vi "Get Section.vi"(10 "sections":string[](array[string]), 11 "info data":string) -> (1 "exist":bool, 3 "section part":string)   [LabVIEW 2013, in "infolib.lvlib"]
doc: "Finds section structure and return its content. If not found, exist is false. If no section structure set, returns whole info data and exist is true."
uses:
  infolib.lvlib
  <vilib>/regexp/Match Regular Expression.xnode
panel:
  out "element":string
  out "regexp":string
  # "testing string: (put \"1\" and \"2\" into section names)"
  # "blfdablad\n#startsection:: 1\njfkdla\n#startsection:: 2\ngroup2group2\n\t  \t#endsection:: 2\njdfkls\n#endsection:: 1\njfdklajfkdl"
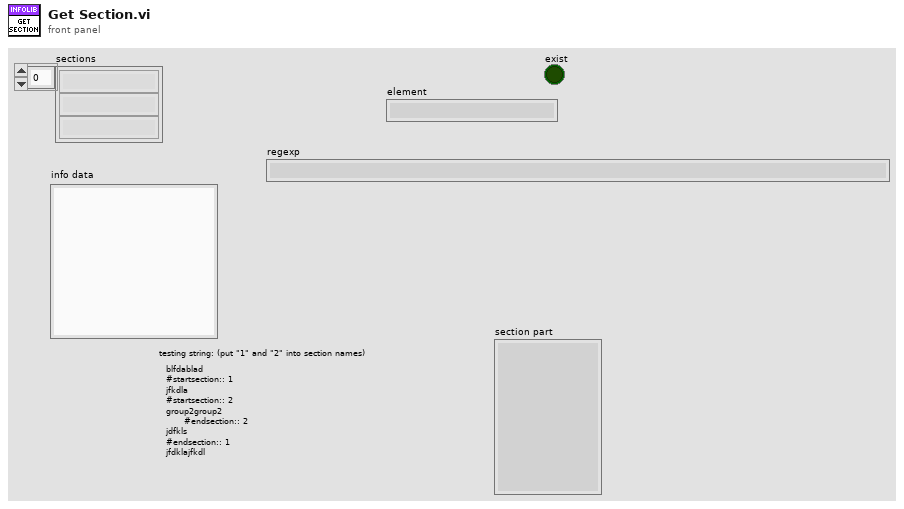
[diagram p1: front panel]
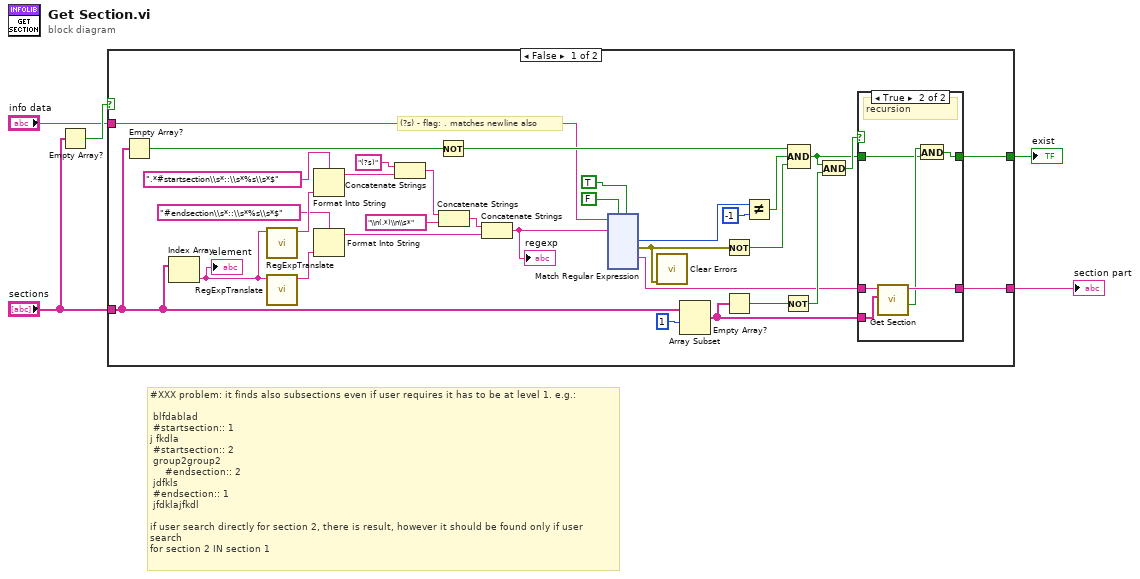
[diagram p0: block diagram]
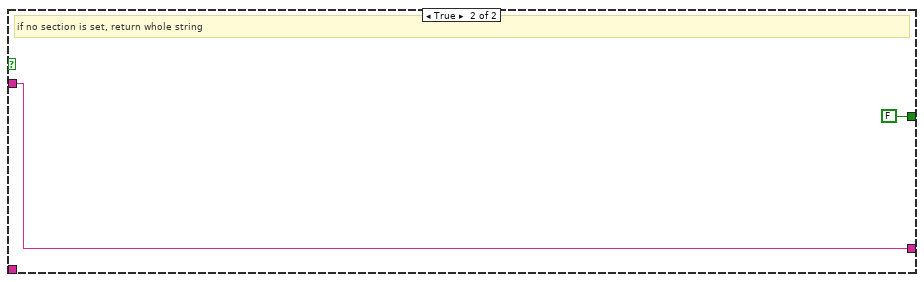
[diagram p3: hidden frame]
diagram:
  # "#XXX problem: it finds also subsections even if user requires it has to be at level 1. e.g.:\n\n blfdablad\n #startsection:: 1\nj fkdla\n #startsection:: 2\n group2group2\n\t   \t#endsection:: 2\n jdfkls\n #endsection:: 1\n jfdklajfkdl\n\nif user search directly for section 2, there is result, however it should be found only if user search\nfor section 2 IN section 1"
  n1 = Empty Array?(array="sections") -> (empty?=w2:bool)
  n2 = case shown="False" w2 {
    tunnel: [w6 FALSE] -> w5
    tunnel: "sections" -> [w15 _]
    tunnel: [w9 w163] -> w3
    tunnel: "info data" -> [w23 w163]
    frame False {
      # "(?s) - flag: . matches newline also"
      n3 = Empty Array?(array=w15) -> (empty?=w28:bool)
      n4 = Index Array(array=w15) -> (element=w16:string)  [unwired: 1 in]
      "element" <- w16
      n5 = call "RegExpTranslate.vi"("string"=w16) -> ("regexp safe string"=w20:string)  [unwired: 10 in]
      n6 = call "RegExpTranslate.vi"("string"=w16) -> ("regexp safe string"=w17:string)  [unwired: 10 in]
      n7 = Format Into String(format string=".*#startsection\\s*::\\s*%s\\s*$", w20) -> (resulting string=w21:string)  [unwired: 2 in, 1 out]
      n8 = Format Into String(format string="#endsection\\s*::\\s*%s\\s*$", w17) -> (resulting string=w18:string)  [unwired: 2 in, 1 out]
      n9 = Concatenate Strings("(?s)" ("section name"), w21) -> (w32:string)
      n10 = Not(x=w28) -> (.not. x?=w27:bool)
      n11 = Concatenate Strings(w32, "\\n(.*)\\n\\s*" ("string")) -> (w30:string)
      n12 = Concatenate Strings(w30, w18) -> (w24:string)
      "regexp" <- w24
      n13 = xnode "Match Regular Expression"("input string"=w23, "regular expression"=w24, "ignore case? (F)"=FALSE, "multiline? (F)"=TRUE) -> ("offset past match"=w34:i32, "error out"=w25:errorcluster, "submatch 1"=w10:string)  [unwired: 2 in, 4 out]
      n14 = call <vilib>:"Clear Errors.vi"("error in (no error)"=w25) -> ()  [unwired: 6 in, 1 out]
      n15 = Array Subset(array=w15, index=1) -> (w8:string[])  [unwired: 1 in]
      n16 = Not(x=w25) -> (.not. x?=w26:bool)
      n17 = Empty Array?(array=w8) -> (empty?=w13:bool)
      n18 = Not Equal?(x=w34, y=-1 ("x")) -> (x != y?=w29:bool)
      n19 = Not(x=w13) -> (.not. x?=w12:bool)
      n20 = Compound Arithmetic op=AND(w27, w29, w26) -> (w7:bool)
      n21 = And(x=w7, y=w12) -> (x .and. y?=w11:bool)
      n22 = case shown="True" w11 {
        tunnel: w10 -> [w39 w45]
        tunnel: [w39 w44] -> w9
        tunnel: w8 -> [_ w43]
        tunnel: w7 -> [w38 w41]
        tunnel: [w38 w40] -> w6
        frame False {
        }
        frame True {
          # "recursion"
          n23 = call "Get Section.vi"("sections"=w43, "info data"=w45) -> ("exist"=w42:bool, "section part"=w44:string)  [unwired: 8 in]
          n24 = And(x=w42, y=w41) -> (x .and. y?=w40:bool)
        }
      }
    }
    frame True {
      # "if no section is set, return whole string"
    }
  }
  "exist" <- w5
  "section part" <- w3
